vi "File Page.vi"(8 "error in (no error)":errorcluster, 11 "Node Ptr":T13 format="%.0x") -> (0 "error out":errorcluster)   [LabVIEW 2015, in "Waveform Data Logger System Explorer.lvlib"]
uses:
  Waveform Data Logger System Explorer.lvlib
  Shared/Types/Boolean Trigger.ctl
  Shared/Types/Value Change Trigger.ctl
  Shared/Types/In Range Trigger.ctl
  Shared/Types/Analog Trigger.ctl
  Shared/Types/Digital Trigger.ctl
  <vilib>/NI Veristand/Custom Device API/Custom Device Item Ref.ctl
  Types/Log Timestamps.ctl
  Shared/Types/Start Trigger.ctl
  Shared/Types/Stop Trigger.ctl
  Shared/Types/Default Trigger.ctl
  Shared/Classes/Log File Specifications/Log File Specification/File Conflict Operation.ctl
  NationalInstruments.VeriStand.SystemStorageUI
  Types/File - Spec Ctl Refs.ctl
  Types/File - Wfm Ctl Refs.ctl
  Types/File - Settings Ctl Refs.ctl
  Types/File - Start Trig Ctl Refs.ctl
  Types/Single Node Browser Data.ctl
  <vilib>/NI Veristand/UI Controls/Single Node Browser/Single Node Browser Ref.ctl
  <vilib>/NI Veristand/UI Controls/Single Node Browser/Callback Type.ctl
  <vilib>/NI Veristand/UI Controls/Single Node Browser/Net Event Data.ctl
  <vilib>/NI Veristand/UI Controls/Single Node Browser/Net Event.ctl
  Types/File - Stop Trig Ctl Refs.ctl
  Types/File Ctl Refs.ctl
  Types/File - Advanced Ctl Refs.ctl
  Types/File - Waveforms.ctl
  <vilib>/Utility/miscctls.llb/LVRowAndColumnUnsignedTypeDef.ctl
  Shared/Types/Trigger Direction.ctl
  <vilib>/NI Veristand/Custom Device API/Get Item Property (Boolean).vi
  Shared/Globals/Property Strings.vi
  <vilib>/NI Veristand/Custom Device API/Set Item Property (Path).vi
  <vilib>/NI Veristand/Custom Device API/Set Item Property (Boolean).vi
  <vilib>/NI Veristand/Custom Device API/Set Item Property (String).vi
  <vilib>/NI Veristand/Custom Device API/Set Item Property (U16).vi
  <vilib>/NI Veristand/Custom Device API/Set Item Property (Double).vi
  <vilib>/NI Veristand/Custom Device API/Set Item Property (U32).vi
  <vilib>/NI VeriStand/Custom Device API/Custom Device API.lvlib
  Shared/Waveform Data Logger Shared.lvlib
  <vilib>/NI VeriStand/UI Controls/Single Node Browser/NI_VS UI Single Node Browser.lvlib
  Shared/Classes/Log File Specifications/Log File Specification/Log File Specification.lvclass
panel:
  in  "Stop Trig":refnum<k24>(container)
  in  "Start Trig":refnum<k24>(container)
  in  "Settings Tab Control":T1(tab)
  in  "File size units":enum16{"MB", "GB"}(ring)=enum."GB"
  in  "File size":dbl=1.0
  in  "SpanMultipleFiles":bool
  in  "Group Name":string
  in  "Use Log As Group Name":bool=TRUE caption="Group Name"
  in  "Log File Path":path=path "c:/logs/{LogName}_{Year}_{Month}_{Day}_{Hour}_{Minute}_{Second}.tdms"
  out "Example Log File Path":path
  in  "File Conflict Operation":T2
  in  "Logged Waveforms":i32[](listbox)
  in  "Select Waveforms":bool
  in  "Retriggerable log":bool
  in  "Start Trig Tab":T3(tab)=enum."Analog"
  in  "Default Start":T4
  in  "Digital Start":T5
  in  "Analog Start":T6
  in  "In Range Start":T7
  in  "Value Change Start":T8
  in  "Boolean Start":T9
  in  "Start trigger channel":string
  in  "Start Trigger":T10 caption="Trigger condition"
  in  "Pre-trig time":dbl=0.5 caption="Pre-trigger duration" format="%#_g seconds"
  in  "Select Start Trig":bool
  in  "Multi Trigs":bool caption="Log multiple triggers simultaneously"
  in  "Stop Trigger":T11 caption="Trigger condition"
  in  "Stop Trig Tab":T3(tab)=enum."Analog"
  in  "Default Stop":T4
  in  "Digital Stop":T5
  in  "Analog Stop":T6
  in  "In Range Stop":T7
  in  "Value Change Stop":T8
  in  "Boolean Stop":T9
  in  "Stop trigger channel":string
  in  "Post-trig time":dbl=0.5 caption="Post-trigger duration" format="%#_g seconds"
  in  "Select Stop Trig":bool
  in  "Log timeout":dbl=2.0 format="%#_g seconds"
  in  "Log timestamps":T12
  in  "CustomBuffer":bool
  in  "MinimumBuffer":u32=1 caption="Minimum Buffer Size"
  in  "Header 2":cluster{"Section Name":string}={"Section Name"="Log File Settings"}
  in  "Header":cluster{"Section Name":string}={"Section Name"="Waveform Log Specification"}
  in  "Description":string
  in  "Name":string
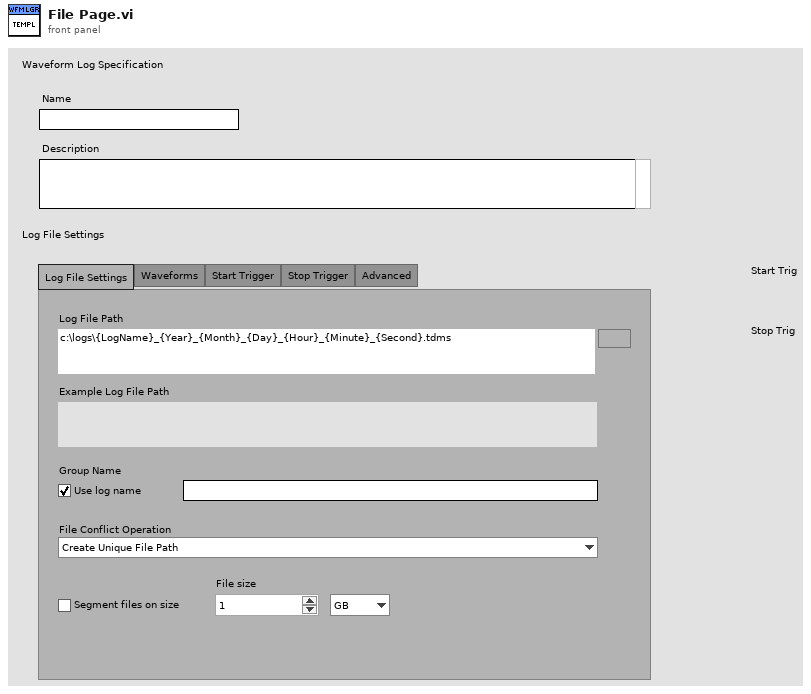
[diagram p1: front panel]
types:
  T1 = enum32{"Log File Settings", "Waveforms", "Start Trigger", "Stop Trigger", "Advanced"}
  T2 = typedef "Waveform Data Logger Shared.lvlib/Log File Specification.lvclass/File Conflict Operation.ctl" = enum16{"Create Unique File Path", "Append to Existing", "Overwrite Existing"}
  T3 = enum32{"Default", "Digital", "Analog", "In Range", "Value Change", "Boolean"}
  T4 = typedef "Waveform Data Logger Shared.lvlib/Default Trigger.ctl" = cluster{"Default State":bool}
  T5 = typedef "Waveform Data Logger Shared.lvlib/Digital Trigger.ctl" = cluster{"Edge":enum16{"Rising", "Falling"}}
  T6 = typedef "Waveform Data Logger Shared.lvlib/Analog Trigger.ctl" = cluster{"Strict edge":bool, "Slope":enum16{"Rising", "Falling"}, "Threshold":dbl}
  T7 = typedef "Waveform Data Logger Shared.lvlib/In Range Trigger.ctl" = cluster{"High limit":dbl, "Low limit":dbl, "Invert?":bool}
  T8 = typedef "Waveform Data Logger Shared.lvlib/Value Change Trigger.ctl" = cluster{"Deadband":dbl}
  T9 = typedef "Waveform Data Logger Shared.lvlib/Boolean Trigger.ctl" = cluster{"Value":dbl, "Operand":enum16{"Equal to", "Not equal to", "Less than", "Less than or equal", "Greater than", "Greater than or equal"}}
  T10 = typedef "Waveform Data Logger Shared.lvlib/Start Trigger.ctl" = enum16{"Start immediately", "Start on digital edge", "Start on analog edge", "Start when in range", "Start when out of range", "Start on value change", "Start when Boolean condition is true"}
  T11 = typedef "Waveform Data Logger Shared.lvlib/Stop Trigger.ctl" = enum16{"Log indefinitely", "Stop after duration", "Stop on digital edge", "Stop on analog edge", "Stop when in range", "Stop when out of range", "Stop on value change", "Stop when Boolean condition is true"}
  T12 = typedef "Waveform Data Logger System Explorer.lvlib/Log Timestamps.ctl" = enum16{"Use waveform timestamps", "Timestamp based on when data is received by the logger"}
  T13 = typedef "Custom Device API.lvlib/Custom Device Item Ref.ctl" = u64
  T14 = typedef "Waveform Data Logger System Explorer.lvlib/File - Advanced Ctl Refs.ctl" = cluster{"Log timeout":refnum<vi>, "Log timestamps":refnum<vi>, "CustomBuffer":refnum<vi>, "MinimumBuffer":refnum<vi>}
  T15 = typedef "Waveform Data Logger System Explorer.lvlib/File Ctl Refs.ctl" = cluster{"File Spec Ctl Refs":T16, "Wfm Ctl Refs":T17, "File Settings Ctl Refs":T18, "Start Trig Ctl Refs":T19, "Stop Trig Ctl Refs":T23, "File Spec Ctl Refs":T14}
  T16 = typedef "Waveform Data Logger System Explorer.lvlib/File - Spec Ctl Refs.ctl" = cluster{"Name":refnum<vi>, "Description":refnum<vi>, "Settings Tab":refnum<vi>}
  T17 = typedef "Waveform Data Logger System Explorer.lvlib/File - Wfm Ctl Refs.ctl" = cluster{"Logged Waveforms":refnum<vi>, "Select Waveforms":refnum<vi>}
  T18 = typedef "Waveform Data Logger System Explorer.lvlib/File - Settings Ctl Refs.ctl" = cluster{"Log File Path":refnum<vi>, "Example Log File Path":refnum<vi>, "Use Log As Group Name":refnum<vi>, "Group Name":refnum<vi>, "File Conflict Operation":refnum<vi>, "SpanMultipleFiles":refnum<vi>, "File size units":refnum<vi>, "File size":refnum<vi>}
  T19 = typedef "Waveform Data Logger System Explorer.lvlib/File - Start Trig Ctl Refs.ctl" = cluster{"Start Trigger":refnum<vi>, "Pre-trig time":refnum<vi>, "Retriggerable log":refnum<vi>, "Multi Trigs":refnum<vi>, "Start trigger channel":refnum<vi>, "Select Start Trig":refnum<vi>, "Start Trig Tab":refnum<vi>, "Default Start":refnum<vi>, "Default State":refnum<vi>, "Digital Start":refnum<vi>, "Analog Start":refnum<vi>, "In Range Start":refnum<vi>, "Invert?":refnum<vi>, "Value Change Start":refnum<vi>, "Boolean Start":refnum<vi>, "Start Trigger .NET":T20}
  T20 = typedef "Waveform Data Logger System Explorer.lvlib/Single Node Browser Data.ctl" = cluster{"ref":T21, "Callbacks":T22}
  T21 = typedef "NI_VS UI Single Node Browser.lvlib/Single Node Browser Ref.ctl" = refnum<k24>
  T22 = typedef "NI_VS UI Single Node Browser.lvlib/Callback Type.ctl" = cluster{"Net Callbacks":refnum<k27>[], "Event":refnum<user-event>}
  T23 = typedef "Waveform Data Logger System Explorer.lvlib/File - Stop Trig Ctl Refs.ctl" = cluster{"Stop Trigger":refnum<vi>, "Post-trig time":refnum<vi>, "Stop trigger channel":refnum<vi>, "Select Stop Trig":refnum<vi>, "Stop Trig Tab":refnum<vi>, "Default Stop":refnum<vi>, "Default State":refnum<vi>, "Digital Stop":refnum<vi>, "Analog Stop":refnum<vi>, "In Range Stop":refnum<vi>, "Invert?":refnum<vi>, "Value Change Stop":refnum<vi>, "Boolean Stop":refnum<vi>, "Stop Trigger .NET":T20}
  T24 = typedef "Custom Device API.lvlib/Custom Device Item Info.ctl" = cluster{"Name":string, "Is Channel":bool, "GUID":string, "Is Waveform":bool}
  T25 = typedef "Waveform Data Logger System Explorer.lvlib/File - Waveforms.ctl" = cluster{"Node Refs":T13[], "Names":string[], "Decimations":u32[]}
  T26 = typedef "LVRowAndColumnUnsignedTypeDef.ctl" = cluster{"Row":u32, "Column":u32}
  T27 = enum8{"Enabled", "Disabled", "Disabled and Grayed Out"}
  T28 = typedef "Waveform Data Logger Shared.lvlib/Trigger Direction.ctl" = enum16{"Start", "Stop"}
  T29 = typedef "Custom Device API.lvlib/Custom Device Commands.ctl" = enum16{"Default", "Item renamed", "Shutdown", "Dynamic button pressed"}
  T30 = typedef "LVRowAndColumnTypeDef.ctl" = cluster{"Row":i32, "Column":i32}
  T31 = typedef "NI_VS UI Single Node Browser.lvlib/Net Event.ctl" = enum16{"SelectedItem"}
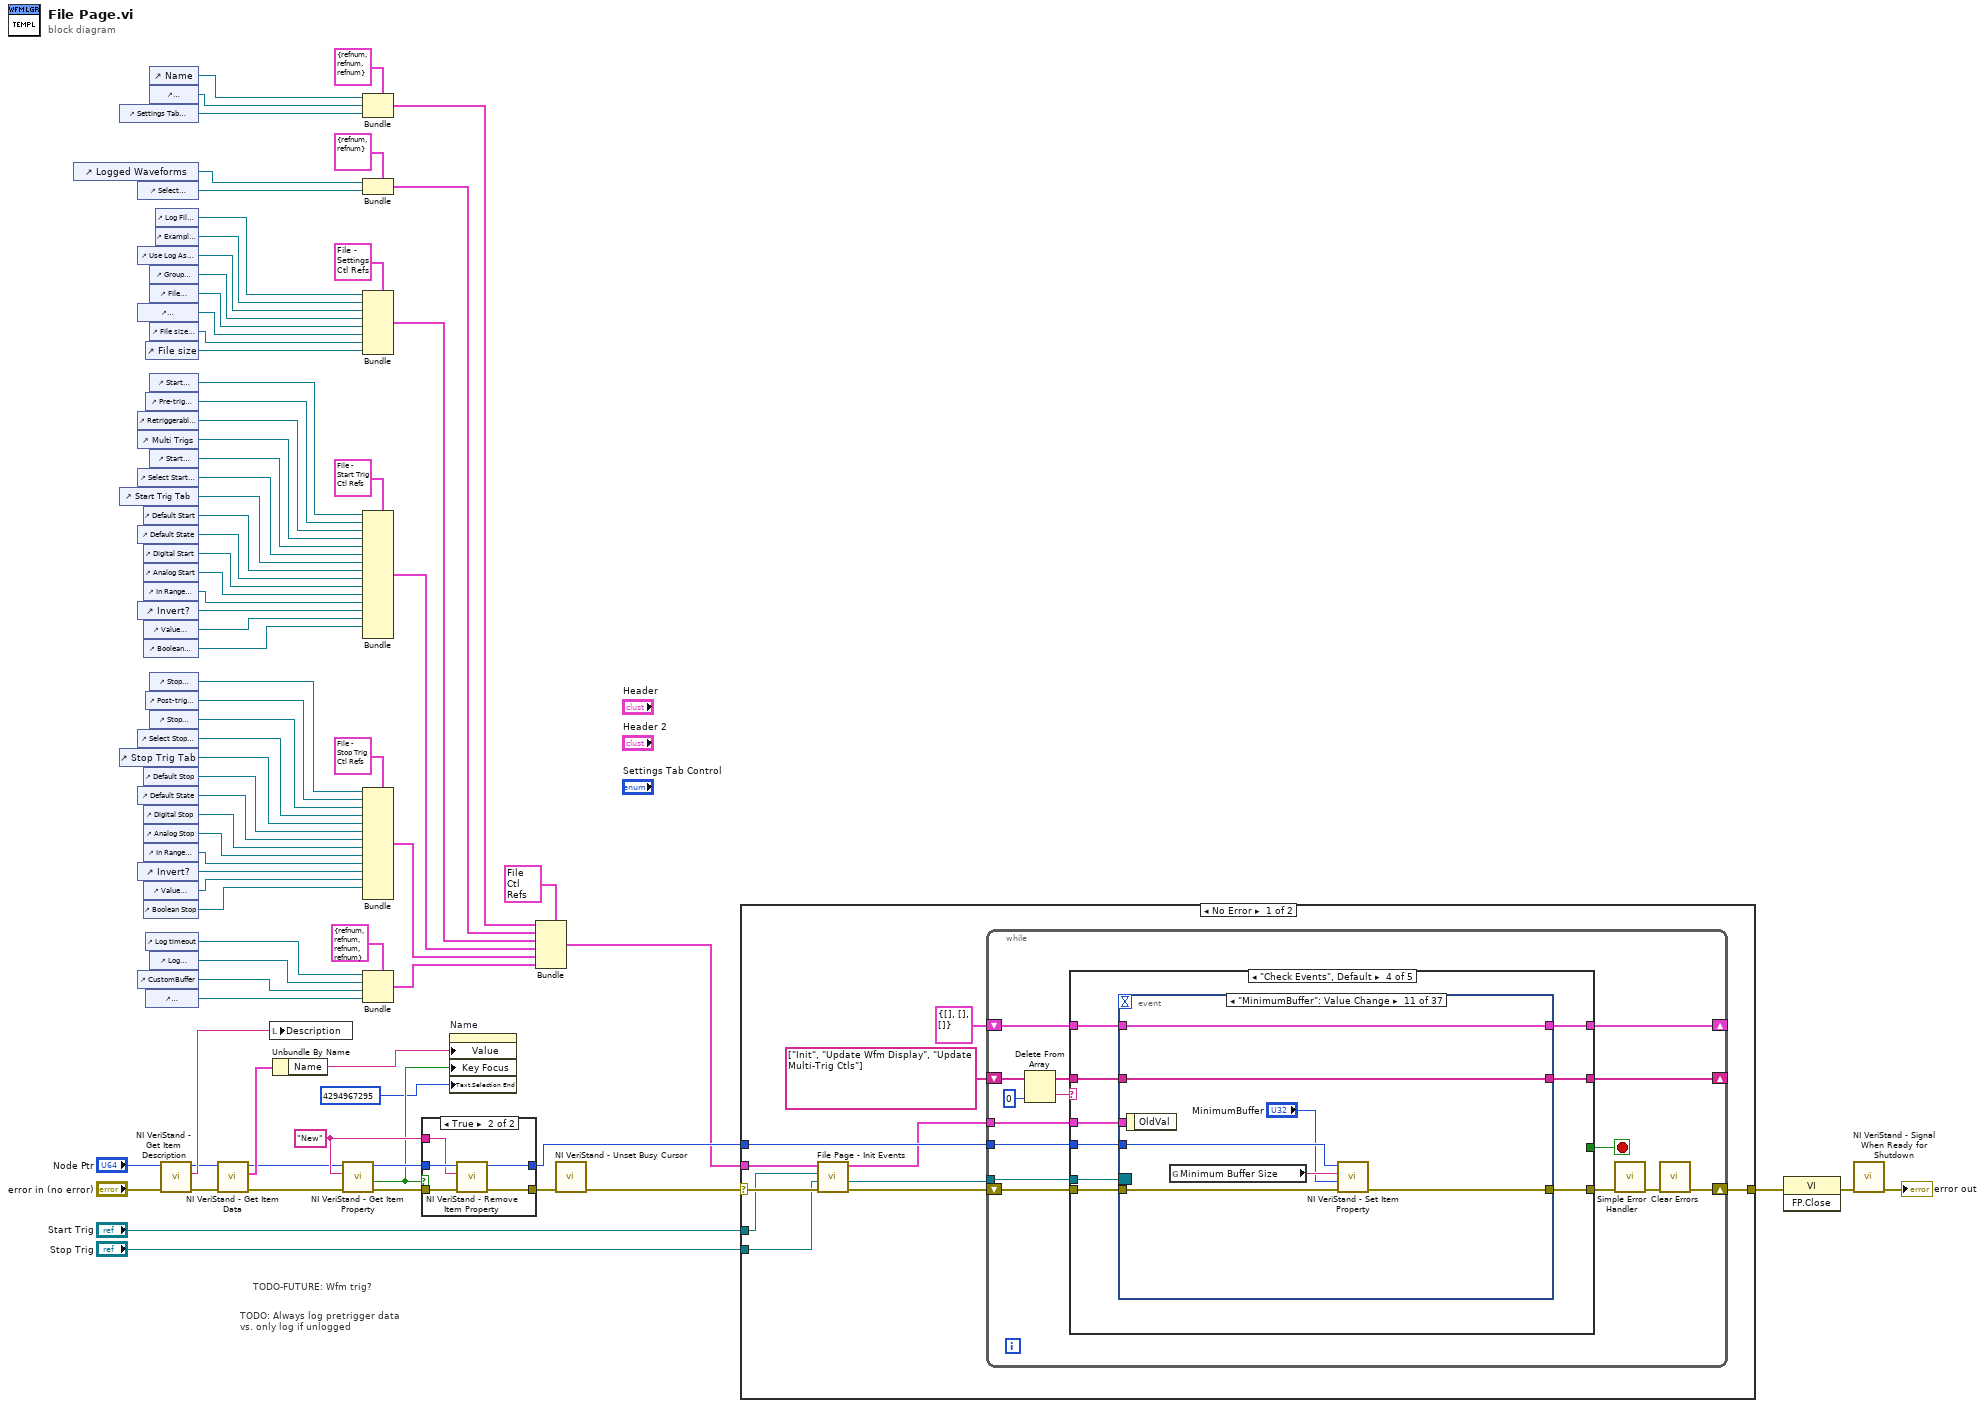
[diagram p0: block diagram]
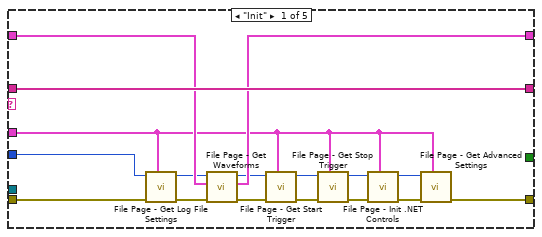
[diagram p3: hidden frame]
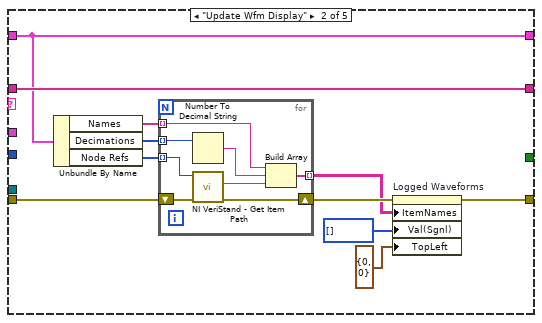
[diagram p4: hidden frame]
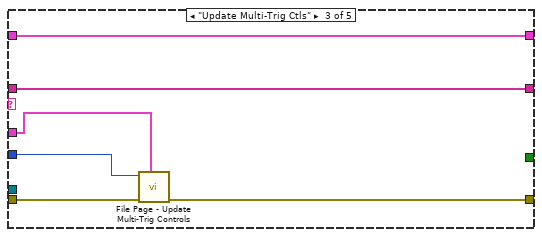
[diagram p5: hidden frame]
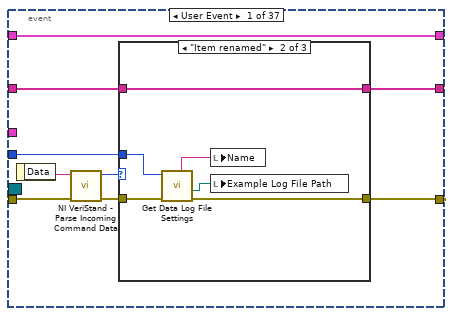
[diagram p6: hidden frame]
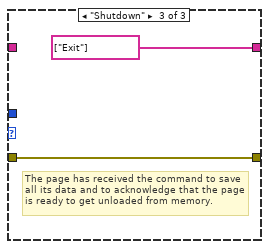
[diagram p8: hidden frame]
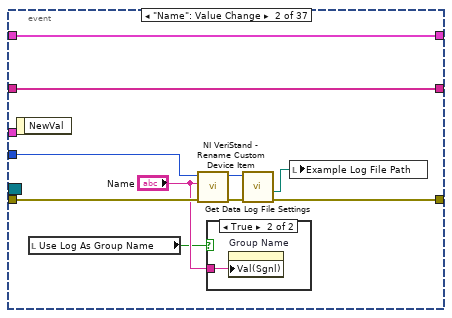
[diagram p9: hidden frame]
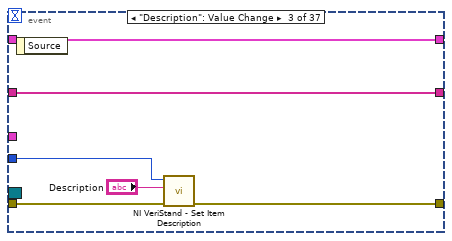
[diagram p11: hidden frame]
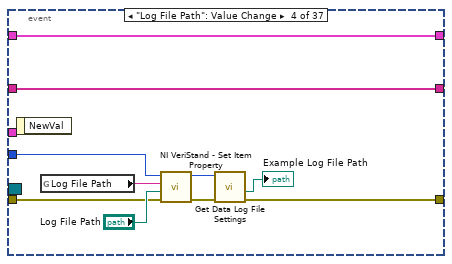
[diagram p12: hidden frame]
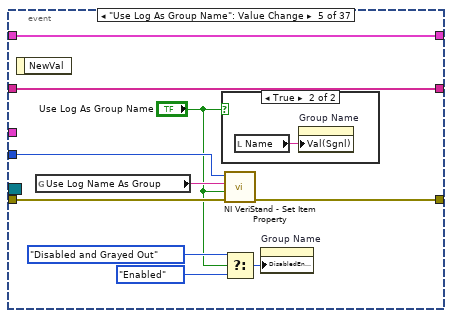
[diagram p13: hidden frame]
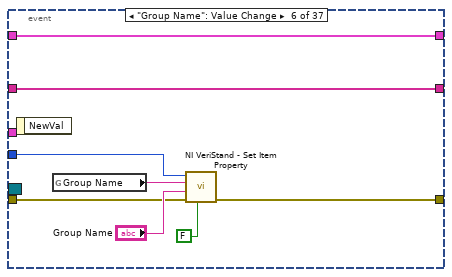
[diagram p15: hidden frame]
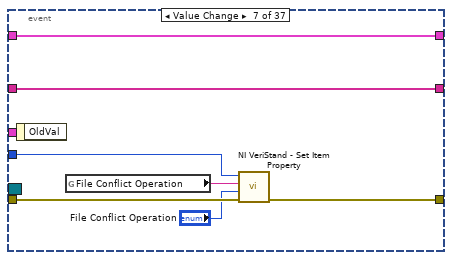
[diagram p16: hidden frame]
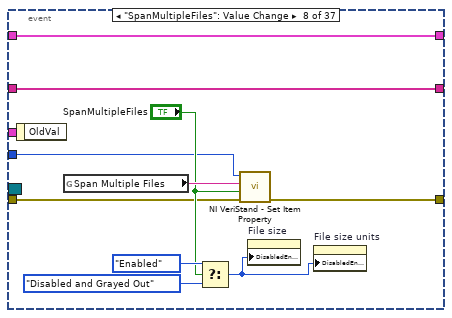
[diagram p17: hidden frame]
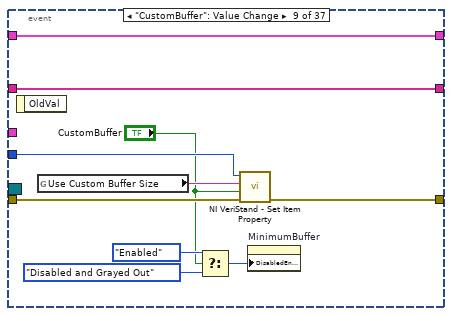
[diagram p18: hidden frame]
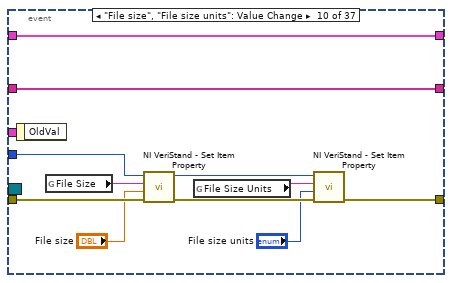
[diagram p19: hidden frame]
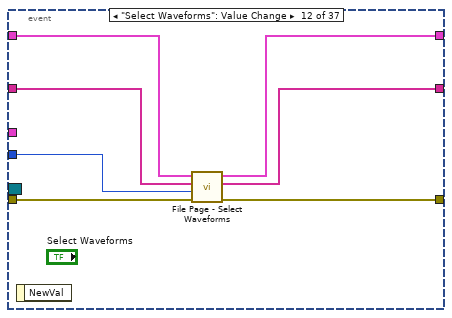
[diagram p20: hidden frame]
diagram:
  w74 = "New" ("Property Name")
  # "TODO: Always log pretrigger data\nvs. only log if unlogged"
  # "TODO-FUTURE: Wfm trig?"
  n1 = control-ref of="Logged Waveforms"() -> (w61:refnum<vi>)
  n2 = control-ref of="Settings Tab Control"() -> (w63:refnum<vi>)
  n3 = control-ref of="Start Trig Tab"() -> (w48:refnum<vi>)
  n4 = control-ref of="Stop Trig Tab"() -> (w39:refnum<vi>)
  n5 = control-ref of="Select Waveforms"() -> (w60:refnum<vi>)
  n6 = control-ref of="Use Log As Group Name"() -> (w53:refnum<vi>)
  n7 = control-ref of="SpanMultipleFiles"() -> (w56:refnum<vi>)
  n8 = control-ref of="Retriggerable log"() -> (w44:refnum<vi>)
  n9 = control-ref of="Multi Trigs"() -> (w45:refnum<vi>)
  n10 = control-ref of="Select Start Trig"() -> (w47:refnum<vi>)
  n11 = control-ref of="Default State"() -> (w23:refnum<vi>)
  n12 = control-ref of="Invert?"() -> (w19:refnum<vi>)
  n13 = control-ref of="Select Stop Trig"() -> (w38:refnum<vi>)
  n14 = control-ref of="Default State"() -> (w16:refnum<vi>)
  n15 = control-ref of="Invert?"() -> (w12:refnum<vi>)
  n16 = control-ref of="CustomBuffer"() -> (w2:refnum<vi>)
  n17 = control-ref of="Default Start"() -> (w49:refnum<vi>)
  n18 = control-ref of="Digital Start"() -> (w22:refnum<vi>)
  n19 = control-ref of="Analog Start"() -> (w21:refnum<vi>)
  n20 = control-ref of="In Range Start"() -> (w20:refnum<vi>)
  n21 = control-ref of="Value Change Start"() -> (w18:refnum<vi>)
  n22 = control-ref of="Boolean Start"() -> (w17:refnum<vi>)
  n23 = control-ref of="Default Stop"() -> (w40:refnum<vi>)
  n24 = control-ref of="Digital Stop"() -> (w15:refnum<vi>)
  n25 = control-ref of="Analog Stop"() -> (w14:refnum<vi>)
  n26 = control-ref of="In Range Stop"() -> (w13:refnum<vi>)
  n27 = control-ref of="Value Change Stop"() -> (w11:refnum<vi>)
  n28 = control-ref of="Boolean Stop"() -> (w10:refnum<vi>)
  n29 = control-ref of="File size"() -> (w58:refnum<vi>)
  n30 = control-ref of="Pre-trig time"() -> (w43:refnum<vi>)
  n31 = control-ref of="Post-trig time"() -> (w36:refnum<vi>)
  n32 = control-ref of="Log timeout"() -> (w32:refnum<vi>)
  n33 = control-ref of="MinimumBuffer"() -> (w1:refnum<vi>)
  n34 = control-ref of="Name"() -> (w65:refnum<vi>)
  n35 = control-ref of="Description"() -> (w64:refnum<vi>)
  n36 = control-ref of="Group Name"() -> (w54:refnum<vi>)
  n37 = control-ref of="File Conflict Operation"() -> (w55:refnum<vi>)
  n38 = control-ref of="File size units"() -> (w57:refnum<vi>)
  n39 = control-ref of="Start Trigger"() -> (w42:refnum<vi>)
  n40 = control-ref of="Start trigger channel"() -> (w46:refnum<vi>)
  n41 = control-ref of="Stop Trigger"() -> (w35:refnum<vi>)
  n42 = control-ref of="Stop trigger channel"() -> (w37:refnum<vi>)
  n43 = control-ref of="Log timestamps"() -> (w33:refnum<vi>)
  n44 = control-ref of="Log File Path"() -> (w51:refnum<vi>)
  n45 = control-ref of="Example Log File Path"() -> (w52:refnum<vi>)
  n46 = call <vilib>:"NI VeriStand - Get Item Description.vi"("error in (no error)"="error in (no error)", "Item Ref in"="Node Ptr") -> ("error out"=w6:errorcluster, "Description"=w77:string, "Item Ref out"=w7:T13)  [unwired: 7 out]
  n47 = call <vilib>:"NI VeriStand - Get Item Data.vi"("error in (no error)"=w6, "Item Ref in"=w7) -> ("error out"=w5:errorcluster, "Item Info"=w9:T24, "Item Ref out"=w4:T13)  [unwired: 7 out]
  n48 = local write "Description"(w77) -> ()
  n49 = Unbundle By Name(w9) -> ("Name"=w8:string)
  n50 = call-poly <vilib>:"NI VeriStand - Get Item Property.vi"("error in (no error)"=w5, "Property Name"=w74, "Item Ref in"=w4) -> ("error out"=w76:errorcluster, "Value"=w71:bool, "Item Ref out"=w75:T13)  [unwired: 5 in, 1 out]
  n51 = Bundle(cluster=T16 {"Name"=refnum, "Description"=refnum, "Settings Tab"=refnum} ("File - Spec Ctl Refs"), "Name"=w65, "Description"=w64, "Settings Tab"=w63) -> (w30:T16)
  n52 = Bundle(cluster=T17 {"Logged Waveforms"=refnum, "Select Waveforms"=refnum} ("Wfm Ctl Refs"), "Logged Waveforms"=w61, "Select Waveforms"=w60) -> (w29:T17)
  n53 = Bundle(cluster=T18 {"Log File Path"=refnum, "Example Log File Path"=refnum, "Use Log As Group Name"=refnum, "Group Name"=refnum, "File Conflict Operation"=refnum, "SpanMultipleFiles"=refnum, "File size units"=refnum, "File size"=refnum} ("File Settings Ctl Refs"), "Log File Path"=w51, "Example Log File Path"=w52, "Use Log As Group Name"=w53, "Group Name"=w54, "File Conflict Operation"=w55, "SpanMultipleFiles"=w56, "File size units"=w57, "File size"=w58) -> (w28:T18)
  n54 = Bundle(cluster=T19 {"Start Trigger"=refnum, "Pre-trig time"=refnum, "Retriggerable log"=refnum, "Multi Trigs"=refnum, "Start trigger channel"=refnum, "Select Start Trig"=refnum, "Start Trig Tab"=refnum, "Default Start"=refnum, "Default State"=refnum, "Digital Start"=refnum, "Analog Start"=refnum, "In Range Start"=refnum, "Invert?"=refnum, "Value Change Start"=refnum, "Boolean Start"=refnum, "Start Trigger .NET"={"ref"=refnum, "Callbacks"={"Net Callbacks"=[], "Event"=refnum}}} ("Start Trig Ctl Refs"), "Start Trigger"=w42, "Pre-trig time"=w43, "Retriggerable log"=w44, "Multi Trigs"=w45, "Start trigger channel"=w46, "Select Start Trig"=w47, "Start Trig Tab"=w48, "Default Start"=w49, "Default State"=w23, "Digital Start"=w22, "Analog Start"=w21, "In Range Start"=w20, "Invert?"=w19, "Value Change Start"=w18, "Boolean Start"=w17) -> (w27:T19)  [unwired: 1 in]
  n55 = Bundle(cluster=T23 {"Stop Trigger"=refnum, "Post-trig time"=refnum, "Stop trigger channel"=refnum, "Select Stop Trig"=refnum, "Stop Trig Tab"=refnum, "Default Stop"=refnum, "Default State"=refnum, "Digital Stop"=refnum, "Analog Stop"=refnum, "In Range Stop"=refnum, "Invert?"=refnum, "Value Change Stop"=refnum, "Boolean Stop"=refnum, "Stop Trigger .NET"={"ref"=refnum, "Callbacks"={"Net Callbacks"=[], "Event"=refnum}}} ("Stop Trig Ctl Refs"), "Stop Trigger"=w35, "Post-trig time"=w36, "Stop trigger channel"=w37, "Select Stop Trig"=w38, "Stop Trig Tab"=w39, "Default Stop"=w40, "Default State"=w16, "Digital Stop"=w15, "Analog Stop"=w14, "In Range Stop"=w13, "Invert?"=w12, "Value Change Stop"=w11, "Boolean Stop"=w10) -> (w26:T23)  [unwired: 1 in]
  n56 = Bundle(cluster=T14 {"Log timeout"=refnum, "Log timestamps"=refnum, "CustomBuffer"=refnum, "MinimumBuffer"=refnum} ("File Spec Ctl Refs"), "Log timeout"=w32, "Log timestamps"=w33, "CustomBuffer"=w2, "MinimumBuffer"=w1) -> (w25:T14)
  n57 = case shown="True" w71 {
    tunnel: w76 -> [w83 w87]
    tunnel: [w83 w84] -> w73
    tunnel: w75 -> [w82 w88]
    tunnel: [w82 w85] -> w72
    tunnel: w74 -> [_ w86]
    frame False {
    }
    frame True {
      n58 = call <vilib>:"NI VeriStand - Remove Item Property.vi"("error in (no error)"=w87, "Property Name"=w86, "Item Ref in"=w88) -> ("error out"=w84:errorcluster, "Item Ref out"=w85:T13)  [unwired: 6 in, 1 out]
    }
  }
  n59 = property on="Name" class="Str"("Value"=w8, "Key Focus"=w71, "Text.Selection End"=u32 4294967295 ("Text.Selection:End")) -> ()  [unwired: 2 in, 2 out]
  n60 = Bundle(cluster=T15 {"File Spec Ctl Refs"={"Name"=refnum, "Description"=refnum, "Settings Tab"=refnum}, "Wfm Ctl Refs"={"Logged Waveforms"=refnum, "Select Waveforms"=refnum}, "File Settings Ctl Refs"={"Log File Path"=refnum, "Example Log File Path"=refnum, "Use Log As Group Name"=refnum, "Group Name"=refnum, "File Conflict Operation"=refnum, "SpanMultipleFiles"=refnum, "File size units"=refnum, "File size"=refnum}, "Start Trig Ctl Refs"={"Start Trigger"=refnum, "Pre-trig time"=refnum, "Retriggerable log"=refnum, "Multi Trigs"=refnum, "Start trigger channel"=refnum, "Select Start Trig"=refnum, "Start Trig Tab"=refnum, "Default Start"=refnum, "Default State"=refnum, "Digital Start"=refnum, "Analog Start"=refnum, "In Range Start"=refnum, "Invert?"=refnum, "Value Change Start"=refnum, "Boolean Start"=refnum, "Start Trigger .NET"={"ref"=refnum, "Callbacks"={"Net Callbacks"=[], "Event"=refnum}}}, "Stop Trig Ctl Refs"={"Stop Trigger"=refnum, "Post-trig time"=refnum, "Stop trigger channel"=refnum, "Select Stop Trig"=refnum, "Stop Trig Tab"=refnum, "Default Stop"=refnum, "Default State"=refnum, "Digital Stop"=refnum, "Analog Stop"=refnum, "In Range Stop"=refnum, "Invert?"=refnum, "Value Change Stop"=refnum, "Boolean Stop"=refnum, "Stop Trigger .NET"={"ref"=refnum, "Callbacks"={"Net Callbacks"=[], "Event"=refnum}}}, "File Spec Ctl Refs"={"Log timeout"=refnum, "Log timestamps"=refnum, "CustomBuffer"=refnum, "MinimumBuffer"=refnum}} ("File Ctl Refs"), "File Spec Ctl Refs"=w30, "Wfm Ctl Refs"=w29, "File Settings Ctl Refs"=w28, "Start Trig Ctl Refs"=w27, "Stop Trig Ctl Refs"=w26, "File Spec Ctl Refs"=w25) -> (w24:T15)
  n61 = call <vilib>:"NI VeriStand - Unset Busy Cursor.vi"("error in (no error)"=w73) -> ("error out"=w78:errorcluster)  [unwired: 10 out]
  n62 = case shown="No Error" w78 {
    selector: w78 -> [w96 w474]
    tunnel: [w97 w472] -> w81
    tunnel: w72 -> [w99 _]
    tunnel: "Stop Trig" -> [w92 _]
    tunnel: "Start Trig" -> [w91 _]
    tunnel: w24 -> [w90 _]
    frame No Error {
      n63 = call "File Page - Init Events.vi"("error in (no error)"=w96, "Stop Trig Ref"=w92, "Start Trig Ref"=w91, "File Ctl Refs in"=w90) -> ("error out"=w95:errorcluster, "Event Registration Refnum"=w94:refnum<event-registration>, "File Ctl Refs out"=w89:T15)  [unwired: 5 in]
      n64 = while {
        tunnel: w99 -> [w112]
        shift-right: [w109] -> w97
        shift-left: w95 -> [w114]
        shift-right: [w103] -> _
        shift-left: string[] ["Init", "Update Wfm Display", "Update Multi-Trig Ctls"] -> [w106]
        tunnel: w94 -> [w108]
        tunnel: w89 -> [w102]
        shift-right: [w100] -> _
        shift-left: T25 {"Node Refs"=[], "Names"=[], "Decimations"=[]} ("File Waveforms") -> [w101]
        stop <- w113 stop-if-true
        n65 = Delete From Array(array=w106, index=0) -> (deleted portion=w105:string, array with subset deleted=w104:string[])  [unwired: 1 in]
        n66 = case shown="\"Check Events\", Default" w105 {
          tunnel: w114 -> [w121 w139 w155 w165 w471]
          tunnel: [_ _ _ _ TRUE] -> w113
          tunnel: w112 -> [w122 _ w156 w164 _]
          tunnel: [w115 w136 w153 w160 w468] -> w111
          tunnel: w108 -> [_ _ _ w163 w466]
          tunnel: w104 -> [w131 w140 w152 w162 w469]
          tunnel: [w131 w140 w152 w161 w469] -> w103
          tunnel: w102 -> [w118 _ w154 w159 w465]
          tunnel: w101 -> [w130 w132 w151 w158 w467]
          tunnel: [w129 w132 w151 w157 w467] -> w100
          frame "Init" {
            n67 = call "File Page - Get Log File Settings.vi"("File Ctl Refs"=w118, "error in (no error)"=w121, "Item Ref in"=w122) -> ("error out"=w124:errorcluster, "Item Ref out"=w123:T13)  [unwired: 7 in]
            n68 = call "File Page - Get Waveforms.vi"("error in (no error)"=w124, "File Waveforms in"=w130, "Item Ref in"=w123) -> ("error out"=w127:errorcluster, "File Waveforms out"=w129:T25, "Item Ref out"=w128:T13)  [unwired: 6 in]
            n69 = call "File Page - Get Start Trigger.vi"("File Ctl Refs"=w118, "error in (no error)"=w127, "Item Ref in"=w128) -> ("error out"=w125:errorcluster, "Item Ref out"=w126:T13)  [unwired: 7 in]
            n70 = call "File Page - Get Stop Trigger.vi"("File Ctl Refs"=w118, "error in (no error)"=w125, "Item Ref in"=w126) -> ("error out"=w119:errorcluster, "Item Ref out"=w120:T13)  [unwired: 7 in]
            n71 = call "File Page - Init .NET Controls.vi"("File Ctl Refs"=w118, "error in (no error)"=w119, "Item Ref in"=w120) -> ("error out"=w117:errorcluster, "Item Ref out"=w116:T13)  [unwired: 7 in]
            n72 = call "File Page - Get Advanced Settings.vi"("File Ctl Refs"=w118, "error in (no error)"=w117, "Item Ref in"=w116) -> ("error out"=w115:errorcluster)  [unwired: 7 in, 1 out]
          }
          frame "Update Wfm Display" {
            n73 = Unbundle By Name(w132) -> ("Names"=w133:string[], "Decimations"=w134:u32[], "Node Refs"=w135:T13[])
            n74 = for {
              shift-right: [w148] -> w138
              shift-left: w139 -> [w150]
              tunnel: w135 -> [w149] mode=indexing
              tunnel: [w146] -> w137 mode=indexing
              tunnel: w133 -> [w143] mode=indexing
              tunnel: w134 -> [w145] mode=indexing
              n75 = Number To Decimal String(number=w145) -> (decimal integer string=w144:string)  [unwired: 1 in]
              n76 = call <vilib>:"NI VeriStand - Get Item Path.vi"("error in (no error)"=w150, "Item Ref in"=w149) -> ("error out"=w148:errorcluster, "Path"=w147:string)  [unwired: 8 out]
              n77 = Build Array(w143, w144, w147) -> (w146:string[])
            }
            n78 = property on="Logged Waveforms" class="MCListbox (strict)"(error in=w138, "ItemNames"=w137, "Val(Sgnl)"=i32[] [] ("Value (Signaling)"), "TopLeft"=T26 {"Row"=0, "Column"=0} ("Top Left Visible Cell")) -> (error out=w136:errorcluster)  [unwired: 1 in, 1 out]
          }
          frame "Update Multi-Trig Ctls" {
            n79 = call "File Page - Update Multi-Trig Controls.vi"("File Ctl Refs in"=w154, "error in (no error)"=w155, "Item Ref in"=w156) -> ("error out"=w153:errorcluster)  [unwired: 8 in]
          }
          frame "Check Events", Default {
            n80 = event shown="[10] \"MinimumBuffer\": Value Change" {
              selector: w163 -> [_ _ _ _ _ _ _ _ _ _ _ _ _ _ _ _ _ _ _ _ _ _ _ _ _ _ _ _ _ _ _ _ _ _ _ _ _]
              dyn-events: _ -> [_ _ _ _ _ _ _ _ _ _ _ _ _ _ _ _ _ _ _ _ _ _ _ _ _ _ _ _ _ _ _ _ _ _ _ _ _]
              timeout: _ -> [_ _ _ _ _ _ _ _ _ _ _ _ _ _ _ _ _ _ _ _ _ _ _ _ _ _ _ _ _ _ _ _ _ _ _ _ _]
              tunnel: w165 -> [w174 w189 w200 w205 w216 w227 w236 w240 w251 w265 w273 w282 w291 w295 w306 w311 w319 w325 w333 w339 w345 w353 w360 w367 w376 w380 w391 w396 w403 w410 w418 w424 w430 w439 w444 w455 w463]
              tunnel: [w170 w194 w199 w211 w214 w226 w233 w239 w250 w261 w270 w279 w290 w293 w304 w310 w316 w324 w332 w338 w344 w351 w358 w366 w375 w379 w389 w395 w399 w408 w415 w423 w429 w437 w443 w454 w459] -> w160
              tunnel: w164 -> [w169 w190 w201 w204 w215 w228 w235 w241 w252 w264 w272 w280 w285 w297 w305 w312 w320 _ w329 w340 w346 w354 w361 w368 w374 w381 w390 _ w400 w411 w417 w425 w431 w438 w446 w456 w464]
              tunnel: w162 -> [w166 w191 w197 w210 w221 w225 w237 w244 w254 w268 w275 w278 w286 _ w303 _ _ w326 w335 w342 w349 w356 w363 w370 w377 _ w388 w397 w406 w413 w420 w427 w434 w441 w448 w457 w458]
              tunnel: [w167 w191 w197 w210 w221 w225 w237 w244 w254 w268 w275 w281 w292 string[] ["Update Multi-Trig Ctls"] w303 string[] ["Update Multi-Trig Ctls"] string[] ["Update Multi-Trig Ctls"] w326 w335 w342 w349 w356 w363 w370 w377 string[] ["Update Multi-Trig Ctls"] w388 w397 w406 w413 w420 w427 w434 w441 w448 w457 w458] -> w161
              tunnel: w159 -> [_ _ _ _ _ _ _ _ _ _ _ _ _ w296 _ _ _ w322 w327 _ _ _ _ _ _ w382 _ w393 w398 _ _ _ _ _ _ _ _]
              tunnel: w158 -> [w168 w185 w196 w202 w213 w223 w231 w238 w249 w258 w271 w277 w287 w299 w300 w308 w315 w321 w334 w336 w343 w350 w357 w364 w371 w384 w385 w392 w405 w407 w414 w421 w428 w435 w442 w449 w460]
              tunnel: [w168 w185 w196 w202 w213 w223 w231 w238 w249 w258 w271 w276 w288 w299 w300 w308 w315 w321 w334 w336 w343 w350 w357 w364 w371 w384 w385 w392 w405 w407 w414 w421 w428 w435 w442 w449 w460] -> w157
              event User Event {
                n81 = event-data() -> ("Data"=w173:string)  [unwired: 1 out]
                n82 = call <vilib>:"NI VeriStand - Parse Incoming Command Data.vi"("error in (no error)"=w174, "Incoming data"=w173) -> ("error out"=w172:errorcluster, "Action"=w171:T29)  [unwired: 8 out]
                n83 = case shown="\"Item renamed\"" w171 {
                  tunnel: w172 -> [w176 w180 w184]
                  tunnel: [w176 w182 w184] -> w170
                  tunnel: w169 -> [_ w181 _]
                  tunnel: [w175 w177 string[] ["Exit"]] -> w167
                  tunnel: w166 -> [w175 w177 _]
                  frame "Default", Default {
                  }
                  frame "Item renamed" {
                    n84 = call "Get Data Log File Settings.vi"("error in"=w180, "File Ref in"=w181) -> ("error out"=w182:errorcluster, "Example File Path"=w178:path, "Name"=w179:string)  [unwired: 7 out]
                    n85 = local write "Name"(w179) -> ()
                    n86 = local write "Example Log File Path"(w178) -> ()
                  }
                  frame "Shutdown" {
                    # "The page has received the command to save all its data and to acknowledge that the page is ready to get unloaded from memory."
                  }
                }
              }
              event "Name": Value Change {
                n87 = event-data() -> ()  [unwired: 2 out]
                n88 = local read "Use Log As Group Name"() -> (w187:bool)
                n89 = call <vilib>:"NI VeriStand - Rename Custom Device Item.vi"("error in (no error)"=w189, "New Name"="Name", "Item Ref in"=w190) -> ("error out"=w193:errorcluster, "Item Ref out"=w192:T13)  [unwired: 1 in, 6 out]
                n90 = case shown="True" w187 {
                  tunnel: "Name" -> [_ w195]
                  frame False {
                  }
                  frame True {
                    n91 = property on="Group Name" class="Str"("Val(Sgnl)"=w195) -> ()  [unwired: 2 in, 2 out]
                  }
                }
                n92 = call "Get Data Log File Settings.vi"("error in"=w193, "File Ref in"=w192) -> ("error out"=w194:errorcluster, "Example File Path"=w186:path)  [unwired: 8 out]
                n93 = local write "Example Log File Path"(w186) -> ()
              }
              event "Description": Value Change {
                n94 = event-data() -> ()  [unwired: 2 out]
                n95 = call <vilib>:"NI VeriStand - Set Item Description.vi"("error in (no error)"=w200, "Description"="Description", "Item Ref in"=w201) -> ("error out"=w199:errorcluster)  [unwired: 8 out]
              }
              event "Log File Path": Value Change {
                n96 = event-data() -> ()  [unwired: 2 out]
                n97 = global read "Property Strings.vi" "Log File Path"() -> (w209:string)
                n98 = call-poly <vilib>:"NI VeriStand - Set Item Property.vi"("error in (no error)"=w205, "Value"="Log File Path", "Property Name"=w209, "Item Ref in"=w204) -> ("error out"=w207:errorcluster, "Item Ref out"=w208:T13)  [unwired: 6 out]
                n99 = call "Get Data Log File Settings.vi"("error in"=w207, "File Ref in"=w208) -> ("error out"=w211:errorcluster, "Example File Path"=→"Example Log File Path":path)  [unwired: 8 out]
              }
              event "Use Log As Group Name": Value Change {
                n100 = event-data() -> ()  [unwired: 2 out]
                n101 = global read "Property Strings.vi" "Use Log Name As Group"() -> (w217:string)
                n102 = case shown="True" "Use Log As Group Name" {
                  frame False {
                  }
                  frame True {
                    n103 = local read "Name"() -> (w222:string)
                    n104 = property on="Group Name" class="Str"("Val(Sgnl)"=w222) -> ()  [unwired: 2 in, 2 out]
                  }
                }
                n105 = call-poly <vilib>:"NI VeriStand - Set Item Property.vi"("error in (no error)"=w216, "Value"="Use Log As Group Name", "Property Name"=w217, "Item Ref in"=w215) -> ("error out"=w214:errorcluster)  [unwired: 5 in, 2 out]
                n106 = Select(t=T27."Disabled and Grayed Out" ("Disabled"), s="Use Log As Group Name", f=T27."Enabled" ("Disabled")) -> (s? t:f=w220:T27)
                n107 = property on="Group Name" class="Str"("DisabledEnum"=w220) -> ()  [unwired: 2 in, 2 out]
              }
              event "Group Name": Value Change {
                n108 = event-data() -> ()  [unwired: 2 out]
                n109 = global read "Property Strings.vi" "Group Name"() -> (w229:string)
                n110 = call-poly <vilib>:"NI VeriStand - Set Item Property.vi"("Binary String (T)"=FALSE, "error in (no error)"=w227, "Value"="Group Name", "Property Name"=w229, "Item Ref in"=w228) -> ("error out"=w226:errorcluster)  [unwired: 4 in, 2 out]
              }
              event Value Change {
                n111 = event-data() -> ()  [unwired: 2 out]
                n112 = global read "Property Strings.vi" "File Conflict Operation"() -> (w234:string)
                n113 = call-poly <vilib>:"NI VeriStand - Set Item Property.vi"("error in (no error)"=w236, "Value"="File Conflict Operation", "Property Name"=w234, "Item Ref in"=w235) -> ("error out"=w233:errorcluster)  [unwired: 5 in, 2 out]
              }
              event "SpanMultipleFiles": Value Change {
                n114 = event-data() -> ()  [unwired: 2 out]
                n115 = global read "Property Strings.vi" "Span Multiple Files"() -> (w243:string)
                n116 = Select(t=T27."Enabled" ("Disabled"), s="SpanMultipleFiles", f=T27."Disabled and Grayed Out" ("Disabled")) -> (s? t:f=w245:T27)
                n117 = call-poly <vilib>:"NI VeriStand - Set Item Property.vi"("error in (no error)"=w240, "Value"="SpanMultipleFiles", "Property Name"=w243, "Item Ref in"=w241) -> ("error out"=w239:errorcluster)  [unwired: 5 in, 2 out]
                n118 = property on="File size" class="DigNum (strict)"("DisabledEnum"=w245) -> ()  [unwired: 2 in, 2 out]
                n119 = property on="File size units" class="Enum (strict)"("DisabledEnum"=w245) -> ()  [unwired: 2 in, 2 out]
              }
              event "CustomBuffer": Value Change {
                n120 = event-data() -> ()  [unwired: 2 out]
                n121 = global read "Property Strings.vi" "Use Custom Buffer Size"() -> (w253:string)
                n122 = Select(t=T27."Enabled" ("Disabled"), s="CustomBuffer", f=T27."Disabled and Grayed Out" ("Disabled")) -> (s? t:f=w255:T27)
                n123 = call-poly <vilib>:"NI VeriStand - Set Item Property.vi"("error in (no error)"=w251, "Value"="CustomBuffer", "Property Name"=w253, "Item Ref in"=w252) -> ("error out"=w250:errorcluster)  [unwired: 5 in, 2 out]
                n124 = property on="MinimumBuffer" class="DigNum (strict)"("DisabledEnum"=w255) -> ()  [unwired: 2 in, 2 out]
              }
              event "File size", "File size units": Value Change {
                n125 = event-data() -> ()  [unwired: 2 out]
                n126 = global read "Property Strings.vi" "File Size"() -> (w267:string)
                n127 = call-poly <vilib>:"NI VeriStand - Set Item Property.vi"("error in (no error)"=w265, "Value"="File size", "Property Name"=w267, "Item Ref in"=w264) -> ("error out"=w262:errorcluster, "Item Ref out"=w263:T13)  [unwired: 5 in, 1 out]
                n128 = global read "Property Strings.vi" "File Size Units"() -> (w266:string)
                n129 = call-poly <vilib>:"NI VeriStand - Set Item Property.vi"("error in (no error)"=w262, "Value"="File size units", "Property Name"=w266, "Item Ref in"=w263) -> ("error out"=w261:errorcluster)  [unwired: 5 in, 2 out]
              }
              event "MinimumBuffer": Value Change {
                n130 = event-data() -> ()  [unwired: 2 out]
                n131 = global read "Property Strings.vi" "Minimum Buffer Size"() -> (w274:string)
                n132 = call-poly <vilib>:"NI VeriStand - Set Item Property.vi"("error in (no error)"=w273, "Value"="MinimumBuffer", "Property Name"=w274, "Item Ref in"=w272) -> ("error out"=w270:errorcluster)  [unwired: 5 in, 2 out]
              }
              event "Select Waveforms": Value Change {
                n133 = event-data() -> ()  [unwired: 2 out]
                n134 = call "File Page - Select Waveforms.vi"("error in (no error)"=w282, "Item Ref in"=w280, "Events in"=w278, "File Waveforms in"=w277) -> ("error out"=w279:errorcluster, "Events out"=w281:string[], "File Waveforms out"=w276:T25)  [unwired: 5 in]
              }
              event "Logged Waveforms": Edit Cell? {
                n135 = event-data() -> ("Coords"=w284:T30, "String"=w283:string)  [unwired: 1 out]
                n136 = call "File Page - Edit Waveform Table.vi"("New String"=w283, "Coords"=w284, "error in (no error)"=w291, "Item Ref in"=w285, "Events in"=w286, "File Waveforms in"=w287) -> ("error out"=w290:errorcluster, "Discard?"=w289:bool, "Events out"=w292:string[], "File Waveforms out"=w288:T25)  [unwired: 2 in]
                n137 = event-data("Discard?"=w289) -> ()  [unwired: 1 in, 1 out]
              }
              event Value Change {
                n138 = event-data() -> ()  [unwired: 2 out]
                n139 = call "File Page - Set Start Trigger.vi"("File Ctl Refs"=w296, "error in (no error)"=w295, "Start Trigger"="Start Trigger", "Item Ref in"=w297) -> ("error out"=w293:errorcluster)  [unwired: 7 in]
              }
              event "Pre-trig time": Value Change {
                n140 = event-data() -> ()  [unwired: 2 out]
                n141 = global read "Property Strings.vi" "Pretrigger Time"() -> (w302:string)
                n142 = call-poly <vilib>:"NI VeriStand - Set Item Property.vi"("error in (no error)"=w306, "Value"="Pre-trig time", "Property Name"=w302, "Item Ref in"=w305) -> ("error out"=w304:errorcluster)  [unwired: 7 out]
              }
              event "Retriggerable log": Value Change {
                n143 = event-data() -> ()  [unwired: 2 out]
                n144 = global read "Property Strings.vi" "Retriggerable"() -> (w313:string)
                n145 = call-poly <vilib>:"NI VeriStand - Set Item Property.vi"("error in (no error)"=w311, "Value"="Retriggerable log", "Property Name"=w313, "Item Ref in"=w312) -> ("error out"=w310:errorcluster)  [unwired: 5 in, 2 out]
              }
              event "Multi Trigs": Value Change {
                n146 = event-data() -> ()  [unwired: 2 out]
                n147 = global read "Property Strings.vi" "Multi Trigs"() -> (w318:string)
                n148 = call-poly <vilib>:"NI VeriStand - Set Item Property.vi"("error in (no error)"=w319, "Value"="Multi Trigs", "Property Name"=w318, "Item Ref in"=w320) -> ("error out"=w316:errorcluster)  [unwired: 5 in, 2 out]
              }
              event "Select Start Trig": Value Change {
                n149 = event-data() -> ()  [unwired: 2 out]
                n150 = Unbundle By Name(w322) -> ("Start Trig Ctl Refs.Start Trigger .NET.ref"=w323:T21)
                n151 = invoke class="NodeBrowserWF" method="ShowDialog"(reference=w323, error in=w325) -> (error out=w324:errorcluster)  [unwired: 1 in, 2 out]
              }
              event User Event {
                n152 = event-data() -> ("Event"=w328:T31, "Data"=w330:variant)  [unwired: 1 out]
                n153 = call "File Page - Select Trigger Channel.vi"("File Ctl Refs"=w327, "Trigger Direction"=Trigger_Direction."Start", "error in (no error)"=w333, "Data"=w330, "Event"=w328, "Item Ref in"=w329) -> ("error out"=w332:errorcluster)  [unwired: 5 in]
              }
              event Value Change {
                n154 = event-data() -> ()  [unwired: 2 out]
                n155 = call "Set Default Trigger.vi"("Trigger Direction"=Trigger_Direction."Start", "error in (no error)"=w339, "Default Trigger"="Default Start", "Item Ref in"=w340) -> ("error out"=w338:errorcluster)  [unwired: 6 in, 1 out]
              }
              event Value Change {
                n156 = event-data() -> ()  [unwired: 2 out]
                n157 = call "Set Digital Trigger.vi"("Trigger Direction"=Trigger_Direction."Start", "error in (no error)"=w345, "Digital Trigger"="Digital Start", "Item Ref in"=w346) -> ("error out"=w344:errorcluster)  [unwired: 6 in, 1 out]
              }
              event Value Change {
                n158 = event-data() -> ()  [unwired: 2 out]
                n159 = call "Set Analog Edge Trigger.vi"("Trigger Direction"=Trigger_Direction."Start", "error in (no error)"=w353, "Analog Trigger"="Analog Start", "Item Ref in"=w354) -> ("error out"=w351:errorcluster)  [unwired: 6 in, 1 out]
              }
              event Value Change {
                n160 = event-data() -> ()  [unwired: 2 out]
                n161 = call "Set In Range Trigger.vi"("Trigger Direction"=Trigger_Direction."Start", "error in (no error)"=w360, "In Range Trigger"="In Range Start", "Item Ref in"=w361) -> ("error out"=w358:errorcluster)  [unwired: 6 in, 1 out]
              }
              event Value Change {
                n162 = event-data() -> ()  [unwired: 2 out]
                n163 = call "Set Value Change Trigger.vi"("Trigger Direction"=Trigger_Direction."Start", "error in (no error)"=w367, "Value Change Trigger"="Value Change Start", "Item Ref in"=w368) -> ("error out"=w366:errorcluster)  [unwired: 6 in, 1 out]
              }
              event Value Change {
                n164 = event-data() -> ()  [unwired: 2 out]
                n165 = call "Set Boolean Trigger.vi"("Trigger Direction"=Trigger_Direction."Start", "error in (no error)"=w376, "Boolean Trigger"="Boolean Start", "Item Ref in"=w374) -> ("error out"=w375:errorcluster)  [unwired: 6 in, 1 out]
              }
              event Value Change {
                n166 = event-data() -> ()  [unwired: 2 out]
                n167 = call "File Page - Set Stop Trigger.vi"("File Ctl Refs"=w382, "error in (no error)"=w380, "Stop Trigger"="Stop Trigger", "Item Ref in"=w381) -> ("error out"=w379:errorcluster)  [unwired: 7 in]
              }
              event "Post-trig time": Value Change {
                n168 = event-data() -> ()  [unwired: 2 out]
                n169 = global read "Property Strings.vi" "Posttrigger Time"() -> (w387:string)
                n170 = call-poly <vilib>:"NI VeriStand - Set Item Property.vi"("error in (no error)"=w391, "Value"="Post-trig time", "Property Name"=w387, "Item Ref in"=w390) -> ("error out"=w389:errorcluster)  [unwired: 7 out]
              }
              event "Select Stop Trig": Value Change {
                n171 = event-data() -> ()  [unwired: 2 out]
                n172 = Unbundle By Name(w393) -> ("Stop Trig Ctl Refs.Stop Trigger .NET.ref"=w394:T21)
                n173 = invoke class="NodeBrowserWF" method="ShowDialog"(reference=w394, error in=w396) -> (error out=w395:errorcluster)  [unwired: 1 in, 2 out]
              }
              event User Event {
                n174 = event-data() -> ("Event"=w401:T31, "Data"=w402:variant)  [unwired: 1 out]
                n175 = call "File Page - Select Trigger Channel.vi"("File Ctl Refs"=w398, "Trigger Direction"=Trigger_Direction."Stop", "error in (no error)"=w403, "Data"=w402, "Event"=w401, "Item Ref in"=w400) -> ("error out"=w399:errorcluster)  [unwired: 5 in]
              }
              event Value Change {
                n176 = event-data() -> ()  [unwired: 2 out]
                n177 = call "Set Default Trigger.vi"("Trigger Direction"=Trigger_Direction."Stop", "error in (no error)"=w410, "Default Trigger"="Default Stop", "Item Ref in"=w411) -> ("error out"=w408:errorcluster)  [unwired: 6 in, 1 out]
              }
              event Value Change {
                n178 = event-data() -> ()  [unwired: 2 out]
                n179 = call "Set Digital Trigger.vi"("Trigger Direction"=Trigger_Direction."Stop", "error in (no error)"=w418, "Digital Trigger"="Digital Stop", "Item Ref in"=w417) -> ("error out"=w415:errorcluster)  [unwired: 6 in, 1 out]
              }
              event Value Change {
                n180 = event-data() -> ()  [unwired: 2 out]
                n181 = call "Set Analog Edge Trigger.vi"("Trigger Direction"=Trigger_Direction."Stop", "error in (no error)"=w424, "Analog Trigger"="Analog Stop", "Item Ref in"=w425) -> ("error out"=w423:errorcluster)  [unwired: 6 in, 1 out]
              }
              event Value Change {
                n182 = event-data() -> ()  [unwired: 2 out]
                n183 = call "Set In Range Trigger.vi"("Trigger Direction"=Trigger_Direction."Stop", "error in (no error)"=w430, "In Range Trigger"="In Range Stop", "Item Ref in"=w431) -> ("error out"=w429:errorcluster)  [unwired: 6 in, 1 out]
              }
              event Value Change {
                n184 = event-data() -> ()  [unwired: 2 out]
                n185 = call "Set Value Change Trigger.vi"("Trigger Direction"=Trigger_Direction."Stop", "error in (no error)"=w439, "Value Change Trigger"="Value Change Stop", "Item Ref in"=w438) -> ("error out"=w437:errorcluster)  [unwired: 6 in, 1 out]
              }
              event Value Change {
                n186 = event-data() -> ()  [unwired: 2 out]
                n187 = call "Set Boolean Trigger.vi"("Trigger Direction"=Trigger_Direction."Stop", "error in (no error)"=w444, "Boolean Trigger"="Boolean Stop", "Item Ref in"=w446) -> ("error out"=w443:errorcluster)  [unwired: 6 in, 1 out]
              }
              event Value Change {
                n188 = event-data() -> ()  [unwired: 2 out]
                n189 = global read "Property Strings.vi" "Ignore timestamps?"() -> (w453:string)
                n190 = Not Equal?(x="Log timestamps", y=Log_Timestamps."Use waveform timestamps" ("Log timestamps")) -> (x != y?=w451:bool)
                n191 = call-poly <vilib>:"NI VeriStand - Set Item Property.vi"("error in (no error)"=w455, "Value"=w451, "Property Name"=w453, "Item Ref in"=w456) -> ("error out"=w454:errorcluster)  [unwired: 7 out]
              }
              event "Log timeout": Value Change {
                n192 = event-data() -> ()  [unwired: 2 out]
                n193 = global read "Property Strings.vi" "Log Timeout"() -> (w462:string)
                n194 = call-poly <vilib>:"NI VeriStand - Set Item Property.vi"("error in (no error)"=w463, "Value"="Log timeout", "Property Name"=w462, "Item Ref in"=w464) -> ("error out"=w459:errorcluster)  [unwired: 7 out]
              }
            }
          }
          frame "Exit" {
            n195 = call "File Page - Exit.vi"("error in (no error)"=w471, "Event Registration Refnum in"=w466, "File Ctl Refs in"=w465) -> ("error out"=w468:errorcluster)  [unwired: 8 in]
          }
        }
        n196 = call <vilib>:"Simple Error Handler.vi"("error in (no error)"=w111) -> ("error out"=w110:errorcluster)  [unwired: 1 in, 7 out]
        n197 = call <vilib>:"Clear Errors.vi"("error in (no error)"=w110) -> ("error out"=w109:errorcluster)  [unwired: 1 in, 5 out]
      }
    }
    frame Error {
      n198 = call <vilib>:"Simple Error Handler.vi"("error in (no error)"=w474) -> ("error out"=w473:errorcluster)  [unwired: 1 in, 7 out]
      n199 = call <vilib>:"Clear Errors.vi"("error in (no error)"=w473) -> ("error out"=w472:errorcluster)  [unwired: 1 in, 5 out]
    }
  }
  n200 = invoke class="VI" method="FP.Close"(error in=w81) -> (error out=w80:errorcluster)  [unwired: 2 in, 2 out]
  n201 = call <vilib>:"NI VeriStand - Signal When Ready for Shutdown.vi"("error in (no error)"=w80) -> ("error out"=→"error out":errorcluster)  [unwired: 10 out]
